vi "Autonomous Independent.vi"() -> ()   [LabVIEW 2013]
doc: "If AutoIDs match then TwoBall? is read from Dashboard, Else it is a control on the Front Panel\n\nINPUTS:\nTwoBall?\nState (Init)\nCollectorArmSpeed\nBrakeDistance\nSlowdownDistance\n\nSTATES:\n\nINIT: Clapper - In, SonicShifter Actuates to Low Gear, RollerPnuematic - Out, Servo - SetAngle (Indicator on Front Panel), IF TwoBall? == True: LowerArm ELSE CheckHotGoal\n\nCHECKHOTGOAL: Runs IsHotGoalDB and puts HotGoal? into Shift Register\n\nLOWERARM: Clapper - OUT, Wait = LowerArmTimeout / 2, RollerPneumatic - WAIT, Collector- LOWER\nWhen Collector has finished or after timeout from LowerArmTimeout and two other timers, Collector - STOP\nIF TwoBall? == TRUE then Collect ELSE Drive12ft\n\nPRECOLLECT: CollectorWrapper - PRECOLLECT\n\nDRIVEBACK: TankDrive -SETVALUE and DriveBackSpeed goes into both desired speeds, Wait - DriveBackWait, TankDrive - SETVALUE and 0 for both desired speeds\n\nCOLLECT: CollectWrapper - COLLECT\n\nSTOPCOLLECT: CollectWrapper - STOP\n\nLIFTARM: Collector - RAISE, Wait - LiftArmWait, Collector - STOP\n\nRAISESERVO: Servo - SETANGLE, Servo takes in RaiseServoAngle from Front Panel\n\nDRIVE12FT: Sonar - READVALUE, AutoDistance - LINEAR, Takes in Drive12ftDistance and distance from the Sonar and BrakeDistance and SlowdownDistance, TankDrive - LINEARDRIVE, Takes in both motor values from AutoDistance and MaxMotorChangeForward/Backward for Desired, TankDrive - LINEARDRIVE, Takes in 0 for Desired and MaxMotorChanges\n\nSHOOT12FT: IF not TwoBall? AND not HotGoal? then Wait - 5500 - ElapsedTime ELSE Pass, Wait - PreShootWait, ShooterWrapper - COLLECTORDOWN\n\nRAISEARM: Wait - PreRaiseArmWait, Collector - RAISE, Takes in CollectorArmSpeed, After Timeout from RaiseArmTimeout or Collector is done , Collector - STOP\n\nSHOOT3FT: Sonar - READVALUE, AutoDistance - LINEAR, Takes in Drive3ftDistance and output form Sonar and Brake/SlowdownDistance, TankDrive - SETVALUE, Takes in AutoDistance values for desired, Exits after AutoDistance is done or Drive3tfTimeout, TankDrive - SETVALUE, Takes in 0 for desired\n\nSHOOT3FT: ShooterWrapper - COLLECTORUP\n\nSTOP: Servo - SETANGLE, 0 for angle"
uses:
  AutoStates.ctl
  Robot Global Data.vi
  SingleSolenoidAction.ctl
  DoubleSolenoidAction.ctl
  ServoAction.ctl
  CollectorAction.ctl
  CollectorWrapAction.ctl
  TankDriveAction.ctl
  AutoAlignMode.ctl
  SonarAction.ctl
  ShooterWrapperAction.ctl
  AutoMode.ctl
  RollerAction.ctl
panel:
  in  "StartShootTime":u32=4500
  in  "SwitchToLowGear?":bool=TRUE
  in  "PreCollectWait":u32=400
  in  "AutoIDKey":i32=3061
  in  "DefaultMotorInput":dbl=0.7
  in  "FarShotMinTime":u32=1000
  in  "CloseShotMinTime":u32=2000
  in  "RotateWait":u32=300
  in  "RotateMotorInput":dbl=0.7
  in  "FarShotDistance":dbl=150.0 format="%#_13g"
  in  "FarShotTimeout":u32=4000
  in  "CloseShotDistance":dbl=36.0 format="%#_13g"
  in  "CloseShotTimeout":u32=4000
  out "CheckGoalTimedOut?":bool
  in  "CheckHotGoalTimeout":u32=1000
  in  "AutoDefaultMode":T1
  in  "ServoInitAngle":i32=140
  in  "RaiseServoAngle":i32=100
  in  "PreShootWait":u32
  in  "MaxMotorChangeBackward":dbl=0.025
  in  "PreRaiseArmWait":u32=500
  in  "MaxMotorChangeForward":dbl=0.05
  out "ElapsedTime":u32
  out "StateTime":u32
  out "CurrentState":T2
  out "RaiseArmTimedOut":bool
  out "Hot?":bool
  out "DriveTimeOut":bool
  out "LowerArmTimedOut":bool
  in  "RaiseArmTimeout":u32=800
  in  "SlowdownDistance":dbl=24.0 format="%#_13g"
  in  "BrakeDistance":dbl=6.0 format="%#_13g"
  in  "CollectorArmSpeed":dbl=1.0 format="%#_13g"
  in  "LiftArmWait":u32=200
  in  "DriveBackWait":u32
  in  "DriveBackSpeed":dbl
  in  "LowerArmTimeout":u32=800
  in  "error in":errorcluster
  out "error out":errorcluster
  # "SHOOT"
  # "SERVO"
  # "HOT GOAL"
  # "OUTPUT"
  # "ROTATE"
  # "GENERAL"
  # "DRIVE"
  # "RAISE/LOWER ARM"
  # "DEPRECATED"
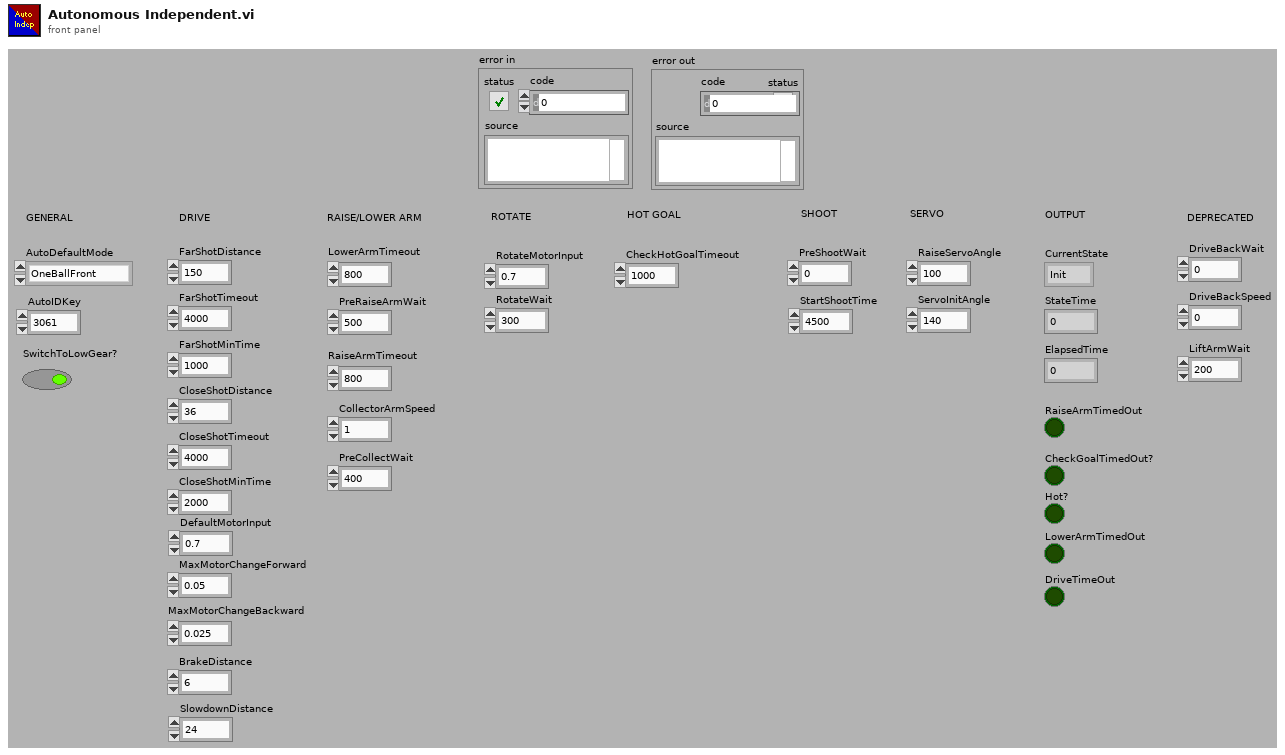
[diagram p1: front panel]
types:
  T1 = typedef "AutoMode.ctl" = enum16{"OneBallFront", "OneBallCollector", "TwoBallNormal", "TwoBallHot"}
  T2 = typedef "AutoStates.ctl" = enum16{"Init", "LowerArmCheckGoal", "DriveBack", "Collect", "StopCollect", "LiftArm", "RaiseServo", "Drive", "Wait", "ShootCollectorUp", "RaiseArm", "ShootCollectorDown", "Rotate1", "Rotate2", "Stop"}
  T3 = typedef "SingleSolenoidAction.ctl" = enum16{"Init", "SetState", "Disable"}
  T4 = typedef "DoubleSolenoidAction.ctl" = enum16{"Init", "Middle", "In", "Out"}
  T5 = typedef "ServoAction.ctl" = enum16{"Init", "SetAngle", "GetAngle", "Lower", "Raise", "Disable"}
  T6 = typedef "CollectorAction.ctl" = enum16{"Init", "Raise", "Lower", "Stop", "GetStatus"}
  T7 = typedef "RollerAction.ctl" = enum16{"Init", "Off", "Forward", "Reverse"}
  T8 = typedef "TankDriveAction.ctl" = enum16{"Init", "LinearDrive", "SetValue", "Disable"}
  T9 = typedef "CollectorWrapAction.ctl" = enum16{"PreCollect", "Collect", "Stop"}
  T10 = typedef "AutoAlignMode.ctl" = enum16{"Fullspeed", "Linear"}
  T11 = typedef "SonarAction.ctl" = enum16{"Init", "ReadValue", "Disable"}
  T12 = typedef "ShooterWrapperAction.ctl" = enum16{"Init", "CollectorDown", "CollectorUp"}
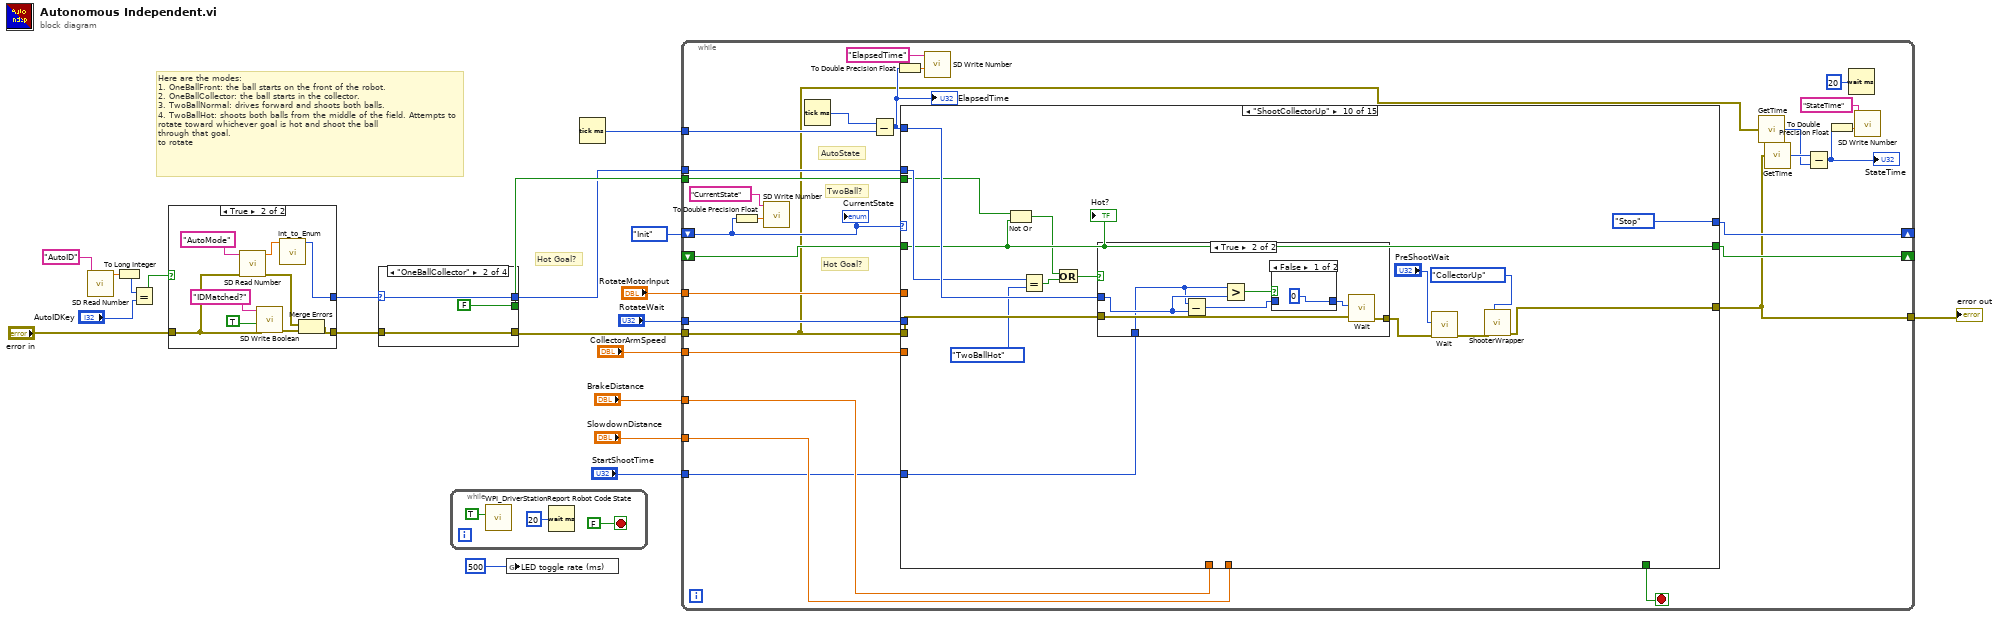
[diagram p0: block diagram]
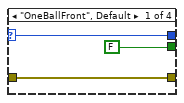
[diagram p2: hidden frame]
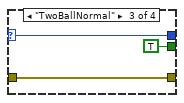
[diagram p3: hidden frame]
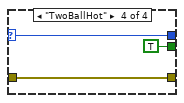
[diagram p4: hidden frame]
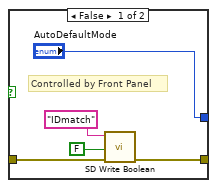
[diagram p5: hidden frame]
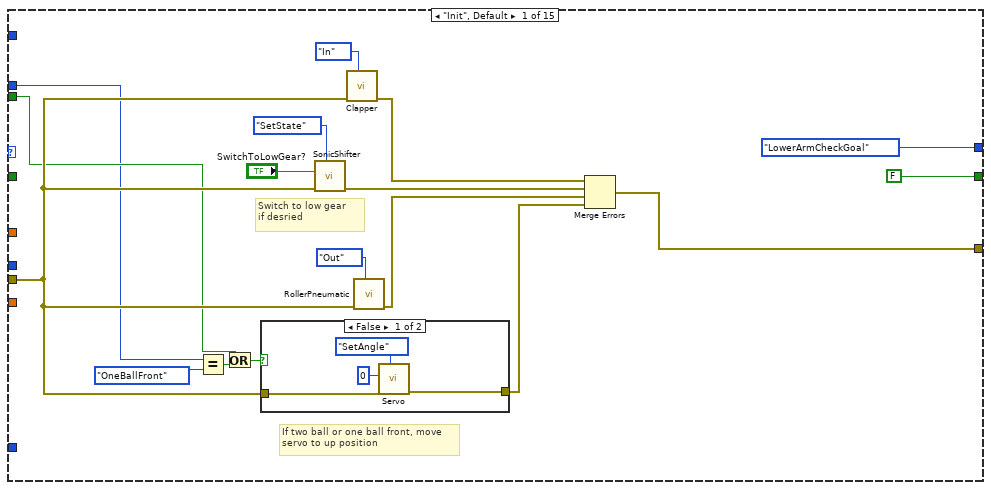
[diagram p6: hidden frame]
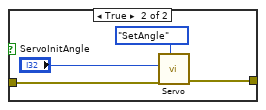
[diagram p7: hidden frame]
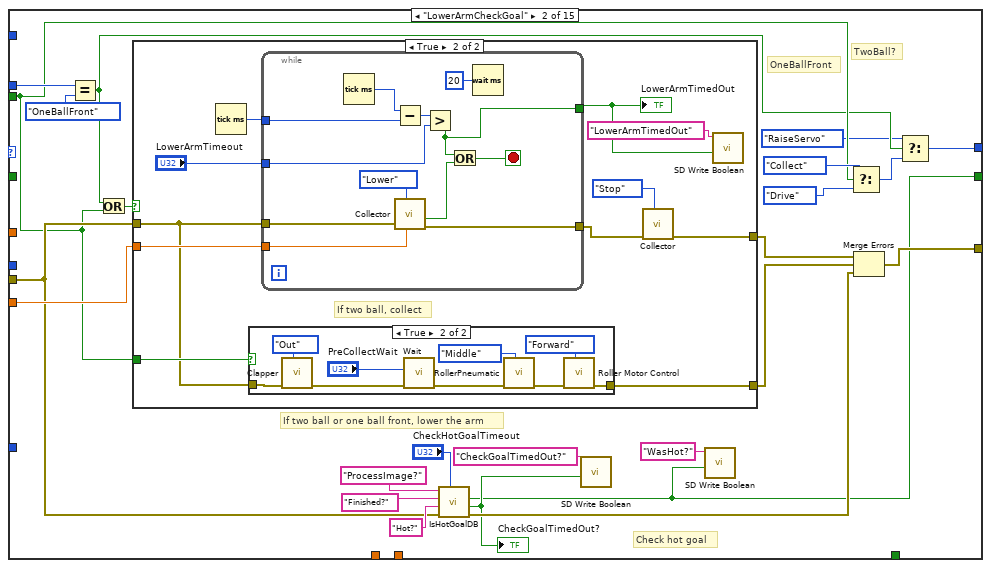
[diagram p8: hidden frame]
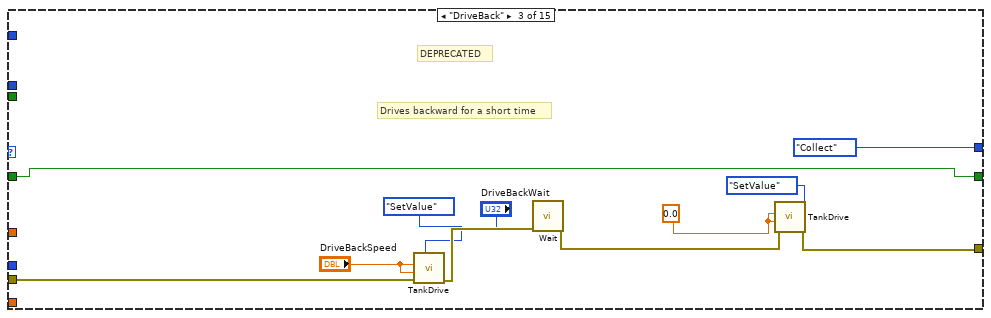
[diagram p11: hidden frame]
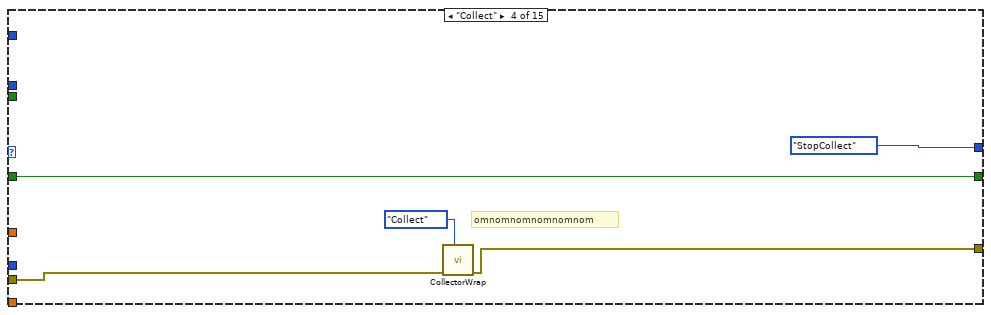
[diagram p12: hidden frame]
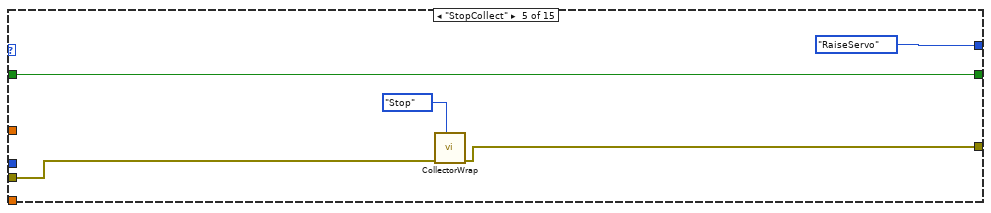
[diagram p13: hidden frame]
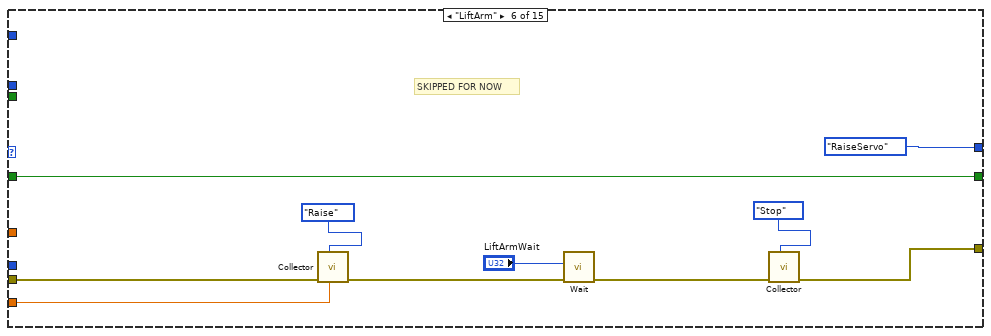
[diagram p14: hidden frame]
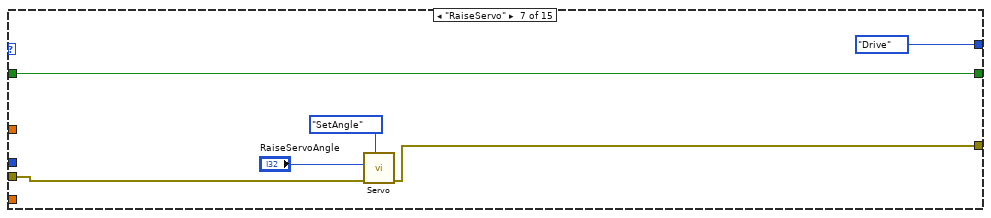
[diagram p15: hidden frame]
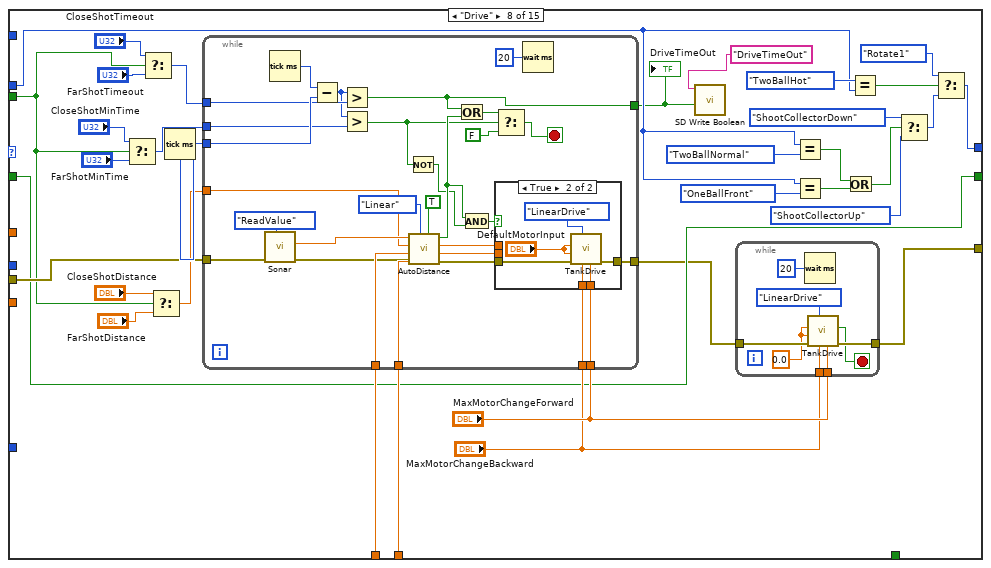
[diagram p16: hidden frame]
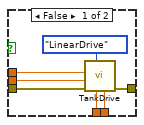
[diagram p17: hidden frame]
diagram:
  # "Here are the modes:\n1. OneBallFront: the ball starts on the front of the robot.\n2. OneBallCollector: the ball starts in the collector.\n3. TwoBallNormal: drives forward and shoots both balls.\n4. TwoBallHot: shoots both balls from the middle of the field. Attempts to rotate toward whichever goal is hot and shoot the ball\nthrough that goal.\nto rotate"
  # "Hot Goal?"
  n1 = call <vilib>:"SD Read Number.vi"("Name"="AutoID") -> ("Numeric"=w20:dbl)  [unwired: 8 in, 2 out]
  n2 = To Long Integer(number=w20) -> (32bit integer=w4:i32)
  n3 = Equal?(x=w4, y="AutoIDKey") -> (x = y?=w13:bool)
  n4 = case shown="True" w13 {
    tunnel: "error in" -> [w25 w33]
    tunnel: [w24 w32] -> w9
    tunnel: ["AutoDefaultMode" w28] -> w11
    frame False {
      # "Controlled by Front Panel"
      n5 = call <vilib>:"SD Write Boolean.vi"("error in"=w25, "Boolean"=FALSE, "Name"="IDmatch") -> ("error out"=w24:errorcluster)  [unwired: 7 in, 1 out]
    }
    frame True {
      n6 = call <vilib>:"SD Read Number.vi"("error in"=w33, "Name"="AutoMode") -> ("error out"=w31:errorcluster, "Numeric"=w29:dbl)  [unwired: 7 in, 1 out]
      n7 = call <vilib>:"SD Write Boolean.vi"("error in"=w33, "Boolean"=TRUE, "Name"="IDMatched?") -> ("error out"=w30:errorcluster)  [unwired: 7 in, 1 out]
      n8 = call "Int_to_Enum.vi"("IntIn"=w29) -> ("EnumOut"=w28:T1)  [unwired: 10 in]
      n9 = Merge Errors(w31, w30) -> (w32:errorcluster)
    }
  }
  n10 = case shown="\"OneBallCollector\"" w11 {
    selector: w11 -> [w36 w39 w42 w45]
    tunnel: [FALSE FALSE TRUE TRUE] -> w10
    tunnel: w9 -> [w37 w40 w43 w46]
    tunnel: [w37 w40 w43 w46] -> w8
    tunnel: [w36 w39 w42 w45] -> w7
    frame "OneBallFront", Default {
    }
    frame "OneBallCollector" {
    }
    frame "TwoBallNormal" {
    }
    frame "TwoBallHot" {
    }
  }
  n11 = while {
    stop <- FALSE stop-if-true
    n12 = call <vilib>:"WPI_DriverStationReport Robot Code State.vi"("Autonomous"=TRUE) -> ()  [unwired: 10 in, 1 out]
    n13 = Wait (ms)(milliseconds to wait=u32 20) -> ()  [unwired: 1 out]
  }
  n14 = global write "Robot Global Data.vi" "LED toggle rate (ms)"(u32 500 ("LED ms toggle rate")) -> ()
  n15 = Tick Count (ms)() -> (millisecond timer value=w14:u32)
  n16 = while {
    shift-right: [w76] -> _
    shift-left: AutoStates."Init" ("Enum") -> [w57]
    shift-right: [w78] -> _
    shift-left: _ -> [w77]
    tunnel: w10 -> [w75]
    tunnel: "CollectorArmSpeed" -> [w73]
    tunnel: "BrakeDistance" -> [w71]
    tunnel: "SlowdownDistance" -> [w72]
    tunnel: w14 -> [w70]
    tunnel: w8 -> [w53]
    tunnel: [w55] -> w21
    tunnel: w7 -> [w67]
    tunnel: "RotateMotorInput" -> [w66]
    tunnel: "RotateWait" -> [w65]
    tunnel: "StartShootTime" -> [w51]
    stop <- w69 stop-if-true
    # "AutoState"
    # "TwoBall?"
    # "Hot Goal?"
    n17 = To Double Precision Float(number=w57) -> (double precision float=w58:dbl)
    n18 = call <vilib>:"SD Write Number.vi"("Numeric"=w58, "Name"="CurrentState") -> ()  [unwired: 8 in, 2 out]
    n19 = Tick Count (ms)() -> (millisecond timer value=w54:u32)
    n20 = Subtract(x=w54, y=w70) -> (x-y=w60:u32)
    "ElapsedTime" <- w60
    n21 = To Double Precision Float(number=w60) -> (double precision float=w59:dbl)
    n22 = case shown="\"ShootCollectorUp\"" w57 {
      selector: w57 -> [_ _ _ _ _ _ _ _ _ _ _ _ _ _ w404]
      tunnel: w53 -> [w87 w121 w172 w177 w182 w187 w197 w231 _ w295 w326 w347 w370 w386 w405]
      tunnel: [w92 w120 w165 w176 w181 w186 w196 w228 _ w297 w324 w352 w365 w385 w399] -> w55
      tunnel: [FALSE ("Hot?") w105 w170 w174 w179 w185 w198 w212 _ w283 w325 w342 w368 w379 w406] -> w78
      tunnel: w77 -> [_ _ w170 w174 w179 w185 w198 w212 _ w283 w325 w342 w368 w379 w406]
      tunnel: [AutoStates."LowerArmCheckGoal" ("Enum") w108 AutoStates."Collect" ("Enum") AutoStates."StopCollect" ("Enum") AutoStates."RaiseServo" ("Enum") AutoStates."RaiseServo" ("Enum") AutoStates."Drive" ("Enum") w210 _ AutoStates."Stop" ("Enum") w310 AutoStates."RaiseArm" ("Enum") AutoStates."ShootCollectorDown" ("Enum") AutoStates."ShootCollectorUp" ("Enum") w404] -> w76
      tunnel: w75 -> [w83 w113 _ _ _ _ _ w201 _ w284 w319 w345 _ _ _]
      tunnel: w73 -> [_ w126 _ _ _ w184 _ _ _ _ w327 _ _ _ _]
      tunnel: w72 -> [_ _ _ _ _ _ _ w230 _ _ _ _ _ _ _]
      tunnel: w71 -> [_ _ _ _ _ _ _ w229 _ _ _ _ _ _ _]
      tunnel: w60 -> [_ _ _ _ _ _ _ _ _ w293 _ w344 _ _ _]
      tunnel: [_ _ _ _ _ _ _ _ _ _ _ _ _ _ TRUE] -> w69
      tunnel: w67 -> [w81 w114 _ _ _ _ _ w208 _ w287 w315 _ _ _ _]
      tunnel: w66 -> [_ _ _ _ _ _ _ _ _ _ _ _ w375 w388 _]
      tunnel: w65 -> [_ _ _ _ _ _ _ _ _ _ _ _ w367 w387 _]
      tunnel: w51 -> [_ _ _ _ _ _ _ _ _ w285 _ w341 _ _ _]
      frame "Init", Default {
        # "If two ball or one ball front, move\nservo to up position"
        # "Switch to low gear\nif desried"
        n23 = Equal?(x=w81, y=AutoMode."OneBallFront") -> (x = y?=w82:bool)
        n24 = Or(x=w83, y=w82) -> (x .or. y?=w84:bool)
        n25 = case shown="False" w84 {
          tunnel: w87 -> [w98 w103]
          tunnel: [w97 w102] -> w90
          frame False {
            n26 = call "Servo.vi"("Action"=ServoAction."SetAngle", "error in (no error)"=w98, "Angle (deg)"=0) -> ("error out"=w97:errorcluster)  [unwired: 7 in, 1 out]
          }
          frame True {
            n27 = call "Servo.vi"("Action"=ServoAction."SetAngle", "error in (no error)"=w103, "Angle (deg)"="ServoInitAngle") -> ("error out"=w102:errorcluster)  [unwired: 7 in, 1 out]
          }
        }
        n28 = call "SonicShifter.vi"("Action"=SingleSolenoidAction."SetState", "error in (no error)"=w87, "Actuate?"="SwitchToLowGear?") -> ("error out"=w88:errorcluster)  [unwired: 8 in]
        n29 = call "Clapper.vi"("State"=DoubleSolenoidAction."In", "Error in"=w87) -> ("Error out"=w89:errorcluster)  [unwired: 9 in]
        n30 = call "RollerPneumatic.vi"("State"=DoubleSolenoidAction."Out", "Error in"=w87) -> ("Error out"=w93:errorcluster)  [unwired: 9 in]
        n31 = Merge Errors(w89, w88, w93, w90) -> (w92:errorcluster)
      }
      frame "LowerArmCheckGoal" {
        # "If two ball or one ball front, lower the arm"
        # "Check hot goal"
        # "OneBallFront"
        # "TwoBall?"
        n32 = Equal?(x=w114, y=AutoMode."OneBallFront") -> (x = y?=w111:bool)
        n33 = Or(x=w111, y=w113) -> (x .or. y?=w116:bool)
        n34 = case shown="True" w116 {
          tunnel: w126 -> [_ w138]
          tunnel: [w128 w137] -> w112
          tunnel: w121 -> [w128 w131]
          tunnel: [w128 w133] -> w117
          tunnel: w113 -> [_ w132]
          frame False {
          }
          frame True {
            # "If two ball, collect"
            n35 = Tick Count (ms)() -> (millisecond timer value=w139:u32)
            n36 = case shown="True" w132 {
              tunnel: [w140 w143] -> w133
              tunnel: w131 -> [w140 w144]
              frame False {
              }
              frame True {
                n37 = call "Clapper.vi"("State"=DoubleSolenoidAction."Out", "Error in"=w144) -> ("Error out"=w148:errorcluster)  [unwired: 9 in]
                n38 = call "Wait.vi"("error in"=w148, "milliseconds to wait"="PreCollectWait") -> ("error out"=w146:errorcluster)  [unwired: 9 in]
                n39 = call "RollerPneumatic.vi"("State"=DoubleSolenoidAction."Middle", "Error in"=w146) -> ("Error out"=w149:errorcluster)  [unwired: 9 in]
                n40 = call "Roller Motor Control.vi"("Action"=RollerAction."Forward", "Error in"=w149) -> ("Error out"=w143:errorcluster)  [unwired: 9 in]
              }
            }
            n41 = while {
              tunnel: w131 -> [w150]
              tunnel: [w161] -> w134
              tunnel: w139 -> [w154]
              tunnel: w138 -> [w153]
              tunnel: [w152] -> w130
              tunnel: "LowerArmTimeout" -> [w151]
              stop <- w156 stop-if-true
              n42 = Tick Count (ms)() -> (millisecond timer value=w158:u32)
              n43 = Subtract(x=w158, y=w154) -> (x-y=w159:u32)
              n44 = call "Collector.vi"("MotorSpeed"=w153, "Action"=CollectorAction."Lower", "Error in"=w150) -> ("Error out"=w161:errorcluster, "Lower Triggered?"=w155:bool)  [unwired: 6 in, 1 out]
              n45 = Greater?(x=w159, y=w151) -> (0:w152:bool)
              n46 = Or(x=w152, y=w155) -> (x .or. y?=w156:bool)
              n47 = Wait (ms)(milliseconds to wait=u32 20) -> ()  [unwired: 1 out]
            }
            "LowerArmTimedOut" <- w130
            n48 = call "Collector.vi"("Action"=CollectorAction."Stop", "Error in"=w134) -> ("Error out"=w137:errorcluster)  [unwired: 7 in, 2 out]
            n49 = call <vilib>:"SD Write Boolean.vi"("Boolean"=w130, "Name"="LowerArmTimedOut") -> ()  [unwired: 8 in, 2 out]
          }
        }
        n50 = call "IsHotGoalDB.vi"("Timeout (ms)"="CheckHotGoalTimeout", "error in"=w121, "DBHot?"="Hot?", "DBFinished?"="Finished?", "DBStart"="ProcessImage?") -> ("error out"=w119:errorcluster, "TimedOut?"=w107:bool, "Hot?"=w105:bool)  [unwired: 4 in]
        "CheckGoalTimedOut?" <- w107
        n51 = call <vilib>:"SD Write Boolean.vi"("Boolean"=w107, "Name"="CheckGoalTimedOut?") -> ()  [unwired: 8 in, 2 out]
        n52 = call <vilib>:"SD Write Boolean.vi"("Boolean"=w105, "Name"="WasHot?") -> ()  [unwired: 8 in, 2 out]
        n53 = Select(t=AutoStates."Collect" ("Enum"), s=w113, f=AutoStates."Drive" ("Enum")) -> (s? t:f=w109:T2)
        n54 = Merge Errors(w112, w117, w119) -> (w120:errorcluster)
        n55 = Select(t=AutoStates."RaiseServo" ("Enum"), s=w111, f=w109) -> (s? t:f=w108:T2)
      }
      frame "DriveBack" {
        w163 = 0.0 ("LeftDesired")
        # "Drives backward for a short time"
        # "DEPRECATED"
        n56 = call "TankDrive.vi"("DriveAction"=TankDriveAction."SetValue", "error in (no error)"=w172, "RightDesired"="DriveBackSpeed", "LeftDesired"="DriveBackSpeed") -> ("error out"=w171:errorcluster)  [unwired: 6 in, 1 out]
        n57 = call "Wait.vi"("error in"=w171, "milliseconds to wait"="DriveBackWait") -> ("error out"=w166:errorcluster)  [unwired: 9 in]
        n58 = call "TankDrive.vi"("DriveAction"=TankDriveAction."SetValue", "error in (no error)"=w166, "RightDesired"=w163, "LeftDesired"=w163) -> ("error out"=w165:errorcluster)  [unwired: 6 in, 1 out]
      }
      frame "Collect" {
        # "omnomnomnomnomnom"
        n59 = call "CollectorWrap.vi"("Action"=CollectorWrapAction."Collect", "error in"=w177) -> ("error out"=w176:errorcluster)  [unwired: 9 in]
      }
      frame "StopCollect" {
        n60 = call "CollectorWrap.vi"("Action"=CollectorWrapAction."Stop", "error in"=w182) -> ("error out"=w181:errorcluster)  [unwired: 9 in]
      }
      frame "LiftArm" {
        # "SKIPPED FOR NOW"
        n61 = call "Collector.vi"("MotorSpeed"=w184, "Action"=CollectorAction."Raise" ("CollectorAction"), "Error in"=w187) -> ("Error out"=w188:errorcluster)  [unwired: 6 in, 2 out]
        n62 = call "Wait.vi"("error in"=w188, "milliseconds to wait"="LiftArmWait") -> ("error out"=w189:errorcluster)  [unwired: 9 in]
        n63 = call "Collector.vi"("Action"=CollectorAction."Stop" ("CollectorAction"), "Error in"=w189) -> ("Error out"=w186:errorcluster)  [unwired: 7 in, 2 out]
      }
      frame "RaiseServo" {
        n64 = call "Servo.vi"("Action"=ServoAction."SetAngle", "error in (no error)"=w197, "Angle (deg)"="RaiseServoAngle") -> ("error out"=w196:errorcluster)  [unwired: 7 in, 1 out]
      }
      frame "Drive" {
        n65 = Select(t="CloseShotMinTime", s=w201, f="FarShotMinTime") -> (s? t:f=w202:u32)
        n66 = Select(t="CloseShotTimeout", s=w201, f="FarShotTimeout") -> (s? t:f=w223:u32)
        n67 = Select(t="CloseShotDistance", s=w201, f="FarShotDistance") -> (s? t:f=w222:dbl)
        n68 = Tick Count (ms)() -> (millisecond timer value=w232:u32)
        n69 = while {
          tunnel: w231 -> [w261]
          tunnel: [w265] -> w205
          tunnel: w232 -> [w266]
          tunnel: w230 -> [w263]
          tunnel: w229 -> [w264]
          tunnel: [w248] -> w200
          tunnel: "MaxMotorChangeForward" -> [w257]
          tunnel: "MaxMotorChangeBackward" -> [w256]
          tunnel: w223 -> [w255]
          tunnel: w222 -> [w254]
          tunnel: w202 -> [w249]
          stop <- w246 stop-if-true
          n70 = call "Sonar.vi"("Action"=SonarAction."ReadValue", "error in (no error)"=w261) -> ("error out"=w258:errorcluster, "distance"=w260:dbl)  [unwired: 8 in]
          n71 = Tick Count (ms)() -> (millisecond timer value=w267:u32)
          n72 = Subtract(x=w267, y=w266) -> (x-y=w250:u32)
          n73 = Greater?(x=w250, y=w255) -> (0:w248:bool)
          n74 = Greater?(x=w250, y=w249) -> (0:w243:bool)
          n75 = Not(x=w243) -> (.not. x?=w242:bool)
          n76 = call "AutoDistance.vi"("Auto"=TRUE, "Mode"=AutoAlignMode."Linear", "Slowdown"=w263, "Brake"=w264, "DesiredDistance"=w254, "CurrentDistance"=w260) -> ("TankDriveRight"=w252:dbl, "TankDriveLeft"=w251:dbl, "Finished"=w244:bool)  [unwired: 3 in]
          n77 = Or(x=w248, y=w244) -> (x .or. y?=w247:bool)
          n78 = And(x=w244, y=w242) -> (x .and. y?=w245:bool)
          n79 = case shown="True" w245 {
            tunnel: [w274 w280] -> w265
            tunnel: w258 -> [w273 w279]
            tunnel: w257 -> [w269 w278]
            tunnel: w256 -> [w270 w277]
            tunnel: w252 -> [w271 _]
            tunnel: w251 -> [w272 _]
            frame False {
              n80 = call "TankDrive.vi"("MaxMotorChangeForward"=w269, "MaxMotorChangeBackwrad"=w270, "DriveAction"=TankDriveAction."LinearDrive", "error in (no error)"=w273, "RightDesired"=w271, "LeftDesired"=w272) -> ("error out"=w274:errorcluster)  [unwired: 4 in, 1 out]
            }
            frame True {
              n81 = call "TankDrive.vi"("MaxMotorChangeForward"=w278, "MaxMotorChangeBackwrad"=w277, "DriveAction"=TankDriveAction."LinearDrive", "error in (no error)"=w279, "RightDesired"="DefaultMotorInput", "LeftDesired"="DefaultMotorInput") -> ("error out"=w280:errorcluster)  [unwired: 4 in, 1 out]
            }
          }
          n82 = Select(t=w247, s=w243, f=FALSE) -> (s? t:f=w246:bool)
          n83 = Wait (ms)(milliseconds to wait=u32 20) -> ()  [unwired: 1 out]
        }
        "DriveTimeOut" <- w200
        n84 = call <vilib>:"SD Write Boolean.vi"("Boolean"=w200, "Name"="DriveTimeOut") -> ()  [unwired: 8 in, 2 out]
        n85 = while {
          tunnel: w205 -> [w240]
          tunnel: [w239] -> w228
          tunnel: "MaxMotorChangeForward" -> [w234]
          tunnel: "MaxMotorChangeBackward" -> [w233]
          stop <- w235 stop-if-true
          w238 = 0.0 ("LeftDesired")
          n86 = Wait (ms)(milliseconds to wait=u32 20) -> ()  [unwired: 1 out]
          n87 = call "TankDrive.vi"("MaxMotorChangeForward"=w234, "MaxMotorChangeBackwrad"=w233, "DriveAction"=TankDriveAction."LinearDrive", "error in (no error)"=w240, "RightDesired"=w238, "LeftDesired"=w238) -> ("error out"=w239:errorcluster, "InRange?"=w235:bool)  [unwired: 4 in]
        }
        n88 = Equal?(x=w208, y=AutoMode."TwoBallNormal") -> (x = y?=w218:bool)
        n89 = Equal?(x=w208, y=AutoMode."OneBallFront") -> (x = y?=w217:bool)
        n90 = Or(x=w218, y=w217) -> (x .or. y?=w213:bool)
        n91 = Equal?(x=AutoMode."TwoBallHot" ("y"), y=w208) -> (x = y?=w207:bool)
        n92 = Select(t=AutoStates."ShootCollectorDown" ("Enum"), s=w213, f=AutoStates."ShootCollectorUp") -> (s? t:f=w211:T2)
        n93 = Select(t=AutoStates."Rotate1" ("Enum"), s=w207, f=w211) -> (s? t:f=w210:T2)
      }
      frame "Wait" {
      }
      frame "ShootCollectorUp" {
        n94 = Not Or(1:w283, 2:w284) -> (0:w282:bool)
        n95 = Equal?(x=w287, y=AutoMode."TwoBallHot") -> (x = y?=w288:bool)
        n96 = Or(x=w282, y=w288) -> (x .or. y?=w289:bool)
        n97 = case shown="True" w289 {
          tunnel: w295 -> [w298 w305]
          tunnel: [w298 w304] -> w294
          tunnel: w293 -> [_ w303]
          tunnel: w285 -> [_ w299]
          frame False {
          }
          frame True {
            n98 = Subtract(x=w299, y=w303) -> (x-y=w300:u32)
            n99 = Greater?(x=w299, y=w303) -> (0:w302:bool)
            n100 = case shown="False" w302 {
              tunnel: [u32 0 w307] -> w301
              tunnel: w300 -> [_ w307]
              frame False {
              }
              frame True {
              }
            }
            n101 = call "Wait.vi"("error in"=w305, "milliseconds to wait"=w301) -> ("error out"=w304:errorcluster)  [unwired: 9 in]
          }
        }
        n102 = call "Wait.vi"("error in"=w294, "milliseconds to wait"="PreShootWait") -> ("error out"=w292:errorcluster)  [unwired: 9 in]
        n103 = call "ShooterWrapper.vi"("Action"=ShooterWrapperAction."CollectorUp", "error in"=w292) -> ("error out"=w297:errorcluster)  [unwired: 8 in]
        "Hot?" <- w283
      }
      frame "RaiseArm" {
        # "Hot Goal?"
        # "TwoBall?"
        # "Give shooter\ntime to come back down"
        n104 = call "Wait.vi"("error in"=w326, "milliseconds to wait"="PreRaiseArmWait") -> ("error out"=w322:errorcluster)  [unwired: 9 in]
        n105 = Tick Count (ms)() -> (millisecond timer value=w328:u32)
        n106 = while {
          tunnel: w322 -> [w340]
          tunnel: [w339] -> w320
          tunnel: w328 -> [w332]
          tunnel: w327 -> [w331]
          tunnel: [w330] -> w309
          stop <- w333 stop-if-true
          n107 = Tick Count (ms)() -> (millisecond timer value=w335:u32)
          n108 = Subtract(x=w335, y=w332) -> (x-y=w336:u32)
          n109 = call "Collector.vi"("MotorSpeed"=w331, "Action"=CollectorAction."Raise", "Error in"=w340) -> ("Error out"=w339:errorcluster, "Upper Triggered?"=w329:bool)  [unwired: 6 in, 1 out]
          n110 = Greater?(x=w336, y="RaiseArmTimeout") -> (0:w330:bool)
          n111 = Wait (ms)(milliseconds to wait=u32 20) -> ()  [unwired: 1 out]
          n112 = Or(x=w330, y=w329) -> (x .or. y?=w333:bool)
        }
        "RaiseArmTimedOut" <- w309
        n113 = call "Collector.vi"("Action"=CollectorAction."Stop", "Error in"=w320) -> ("Error out"=w324:errorcluster)  [unwired: 7 in, 2 out]
        n114 = call <vilib>:"SD Write Boolean.vi"("Boolean"=w309, "Name"="RaiseArmTimedOut") -> ()  [unwired: 8 in, 2 out]
        n115 = Equal?(x=w315, y=AutoMode."TwoBallHot") -> (x = y?=w313:bool)
        n116 = Not(x=w319) -> (.not. x?=w318:bool)
        n117 = Select(t=AutoStates."Stop" ("Enum"), s=w318, f=AutoStates."ShootCollectorUp" ("Enum")) -> (s? t:f=w311:T2)
        n118 = Select(t=AutoStates."Rotate2" ("Enum"), s=w313, f=w311) -> (s? t:f=w310:T2)
      }
      frame "ShootCollectorDown" {
        # "AND"
        # "001\n111\n010\n100"
        n119 = Not(x=w345) -> (.not. x?=w349:bool)
        n120 = Not(x=w342) -> (.not. x?=w348:bool)
        n121 = And(x=w349, y=w348) -> (x .and. y?=w343:bool)
        n122 = case shown="True" w343 {
          tunnel: w347 -> [w353 w360]
          tunnel: [w353 w359] -> w346
          tunnel: w344 -> [_ w358]
          tunnel: w341 -> [_ w354]
          frame False {
          }
          frame True {
            n123 = Subtract(x=w354, y=w358) -> (x-y=w355:u32)
            n124 = Greater?(x=w354, y=w358) -> (0:w357:bool)
            n125 = case shown="False" w357 {
              tunnel: [u32 0 w362] -> w356
              tunnel: w355 -> [_ w362]
              frame False {
              }
              frame True {
              }
            }
            n126 = call "Wait.vi"("error in"=w360, "milliseconds to wait"=w356) -> ("error out"=w359:errorcluster)  [unwired: 9 in]
          }
        }
        n127 = call "ShooterWrapper.vi"("Action"=ShooterWrapperAction."CollectorDown", "error in"=w346) -> ("error out"=w352:errorcluster)  [unwired: 8 in]
      }
      frame "Rotate1" {
        w364 = 0.0
        # "ASSUME CAMERA POINTED LEFT"
        n128 = Select(t=1.0, s=w368, f=-1.0) -> (s? t:f=w377:dbl)
        n129 = Multiply(x=w377, y=w375) -> (x*y=w374:dbl)
        n130 = Negate(x=w374) -> (-x=w373:dbl)
        n131 = call "TankDrive.vi"("DriveAction"=TankDriveAction."SetValue", "error in (no error)"=w370, "RightDesired"=w374, "LeftDesired"=w373) -> ("error out"=w369:errorcluster)  [unwired: 6 in, 1 out]
        n132 = call "Wait.vi"("error in"=w369, "milliseconds to wait"=w367) -> ("error out"=w366:errorcluster)  [unwired: 9 in]
        n133 = call "TankDrive.vi"("DriveAction"=TankDriveAction."SetValue", "error in (no error)"=w366, "RightDesired"=w364, "LeftDesired"=w364) -> ("error out"=w365:errorcluster)  [unwired: 6 in, 1 out]
      }
      frame "Rotate2" {
        w390 = 0.0
        n134 = Select(t=1.0, s=w379, f=-1.0) -> (s? t:f=w395:dbl)
        n135 = Multiply(x=w395, y=w388) -> (x*y=w384:dbl)
        n136 = Negate(x=w384) -> (-x=w383:dbl)
        n137 = call "TankDrive.vi"("DriveAction"=TankDriveAction."SetValue", "error in (no error)"=w386, "RightDesired"=w383, "LeftDesired"=w384) -> ("error out"=w392:errorcluster)  [unwired: 6 in, 1 out]
        n138 = Multiply(x=u32 2, y=w387) -> (x*y=w382:u32)
        n139 = call "Wait.vi"("error in"=w392, "milliseconds to wait"=w382) -> ("error out"=w391:errorcluster)  [unwired: 9 in]
        n140 = call "TankDrive.vi"("DriveAction"=TankDriveAction."SetValue", "error in (no error)"=w391, "RightDesired"=w390, "LeftDesired"=w390) -> ("error out"=w385:errorcluster)  [unwired: 6 in, 1 out]
      }
      frame "Stop" {
        n141 = call "Servo.vi"("Action"=ServoAction."SetAngle", "error in (no error)"=w405, "Angle (deg)"=0) -> ("error out"=w402:errorcluster)  [unwired: 7 in, 1 out]
        n142 = call "SonicShifter.vi"("Action"=SingleSolenoidAction."SetState", "error in (no error)"=w402, "Actuate?"=FALSE) -> ("error out"=w399:errorcluster)  [unwired: 8 in]
      }
    }
    n143 = call <vilib>:"SD Write Number.vi"("Numeric"=w59, "Name"="ElapsedTime") -> ()  [unwired: 8 in, 2 out]
    n144 = call "GetTime.vi"("error in"=w53) -> ("Time"=w52:u32)
    n145 = call "GetTime.vi"("error in"=w55) -> ("Time"=w68:u32)
    n146 = Subtract(x=w68, y=w52) -> (x-y=w64:u32)
    "StateTime" <- w64
    n147 = To Double Precision Float(number=w64) -> (double precision float=w62:dbl)
    n148 = Wait (ms)(milliseconds to wait=u32 20) -> ()  [unwired: 1 out]
    n149 = call <vilib>:"SD Write Number.vi"("Numeric"=w62, "Name"="StateTime") -> ()  [unwired: 8 in, 2 out]
    "CurrentState" <- w57
  }
  "error out" <- w21
